vi "Init.vi"(8 "error in (no error)":errorcluster, 11 "Tree in":refnum<vi>) -> (0 "error out":errorcluster, 3 "Tree out":refnum<vi>)   [LabVIEW 2019, in "BlueVariantView.lvlib"]
doc: "This method initializes your tree control.\nYou only need to call this method once.\nThis will apply custom symbols to the tree reference"
uses:
  BlueVariantView.lvlib
  Defer Panel Updates/Defer Panel Updates BVV.lvlib
  Defer Panel Updates/SubVIs/defer panel updates Controlref step1.vi
  Defer Panel Updates/SubVIs/defer panel updates step2.vi
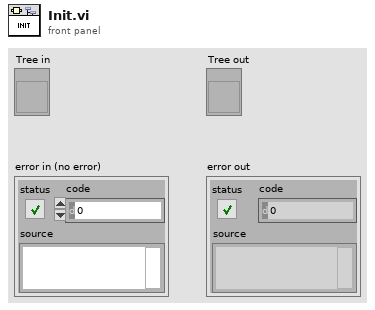
[diagram p1: front panel]
types:
  T1 = typedef "Defer Panel Updates BVV.lvlib/defer panel updates data.ctl" = cluster{"Owning VI":refnum<vi>, "Front Panel":refnum<vi>, "performed?":bool}
  T2 = cluster{"image type":i32, "image depth":i32, "image":u8[], "mask":u8[], "colors":u32[], "Rectangle":cluster{"left":i16, "top":i16, "right":i16, "bottom":i16}}[]
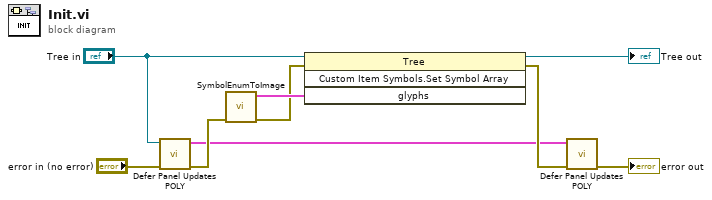
[diagram p0: block diagram]
diagram:
  n1 = call-poly "Defer Panel Updates POLY.vi"("error in (no error)"="error in (no error)", "control reference"="Tree in") -> ("error out"=w4:errorcluster, "Refs"=w1:T1)  [unwired: 8 in]
  n2 = call "SymbolEnumToImage.vi"("error in (no error)"=w4) -> ("error out"=w8:errorcluster, "Symbols"=w9:T2)  [unwired: 9 in]
  n3 = invoke class="Tree" method="Custom Item Symbols.Set Symbol Array"(reference="Tree in", error in=w8, "glyphs"=w9) -> (reference out=→"Tree out":refnum<vi>, error out=w3:errorcluster)  [unwired: 1 in, 2 out]
  n4 = call-poly "Defer Panel Updates POLY.vi"("error in (no error)"=w3, "Refs"=w1) -> ("error out"=→"error out":errorcluster)  [unwired: 9 in]
